vi "RT-all停止全局.vi"() -> ()   [LabVIEW 2013]
panel:
  out "RT-all停止":bool
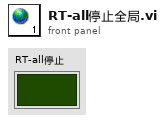
[diagram p1: front panel]
diagram:
